vi "Read.vi"(8 "error in (no error)":errorcluster, 11 "Bronkhorst Settings in":T1) -> (0 "error out":errorcluster, 1 "Connection Error":bool, 2 "flow":dbl, 3 "Bronkhorst Settings out":T1)   [LabVIEW 2018, in "Bronkhorst M13 Flow Meter.lvlib"]
uses:
  Bronkhorst M13 Flow Meter.lvlib
  Settings Cluster.ctl
  <vilib>/regexp/Match Regular Expression.xnode
  <vilib>/ptbypt/NI_PtbyPt.lvlib
panel:
  out "x/y":dbl
  out "whole match":string
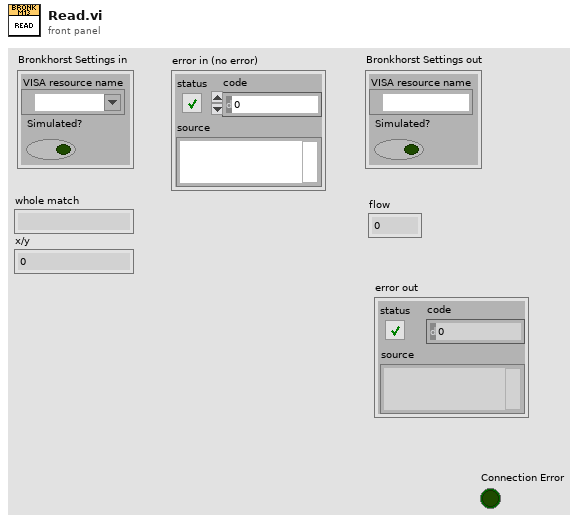
[diagram p1: front panel]
types:
  T1 = typedef "Bronkhorst M13 Flow Meter.lvlib/Settings Cluster.ctl" = cluster{"VISA resource name":refnum<visa-resource-name>, "Simulated?":bool}
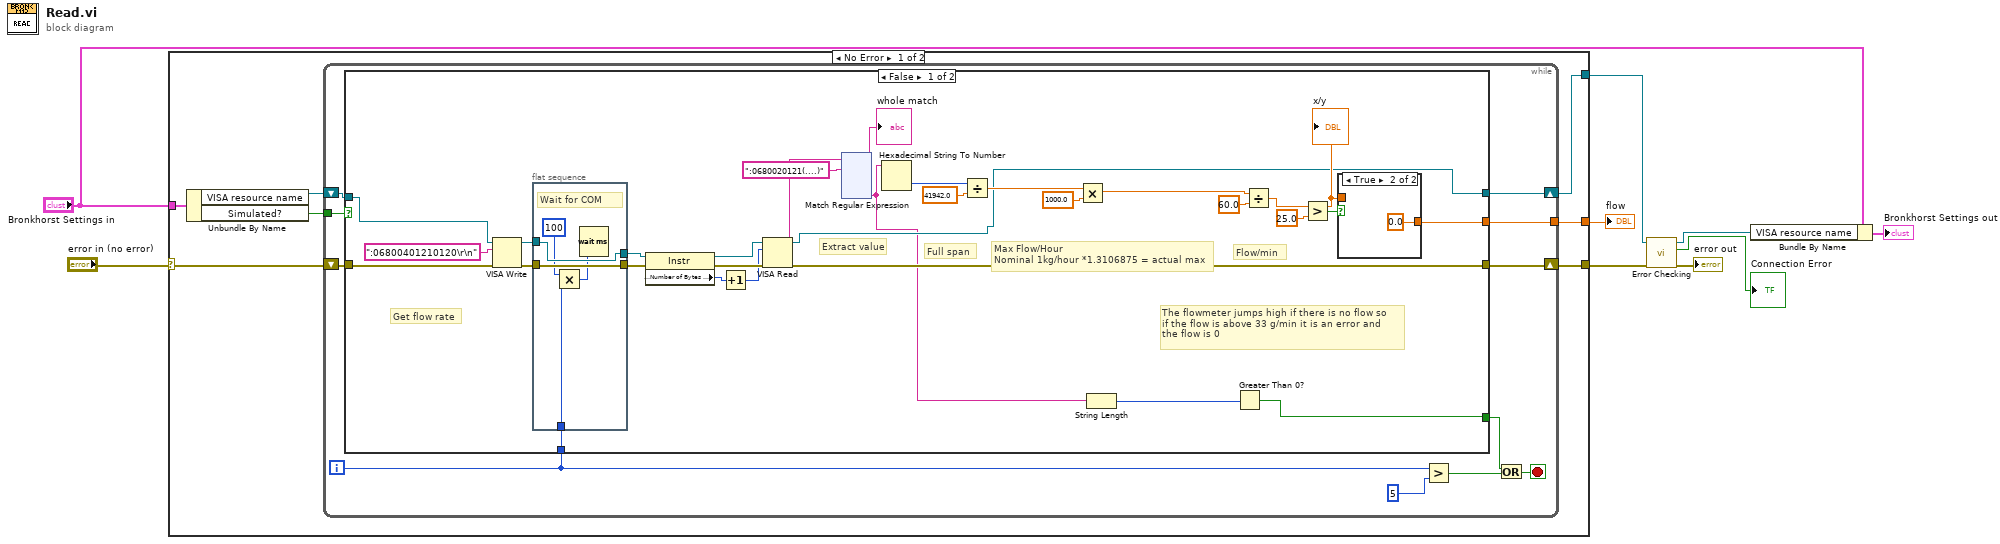
[diagram p0: block diagram]
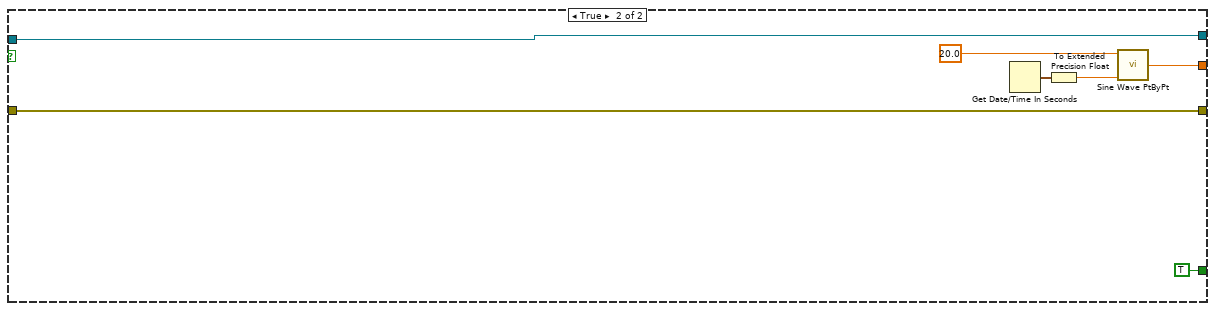
[diagram p3: hidden frame]
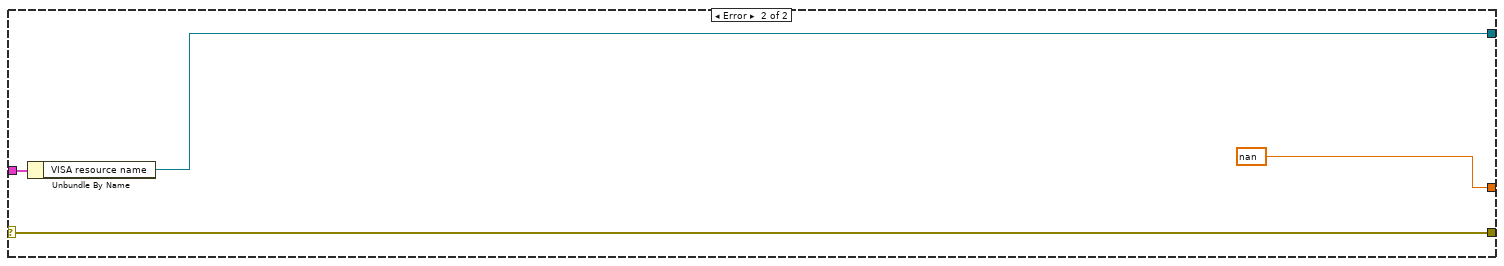
[diagram p4: hidden frame]
diagram:
  n1 = case shown="No Error" "error in (no error)" {
    selector: "error in (no error)" -> [w15 w191]
    tunnel: [w14 w191] -> w3
    tunnel: "Bronkhorst Settings in" -> [w12 w189]
    tunnel: [w13 nan ("sine wave")] -> w9
    tunnel: [w10 w188] -> w5
    frame No Error {
      n2 = Unbundle By Name(w12) -> ("VISA resource name"=w11:refnum<visa-resource-name>, "Simulated?"=w16:bool)
      n3 = while {
        tunnel: w16 -> [w27]
        tunnel: [w24] -> w13
        shift-right: [w25] -> w14
        shift-left: w15 -> [w26]
        shift-right: [w22] -> w10
        shift-left: w11 -> [w23]
        i -> [w18]
        stop <- w17 stop-if-true
        n4 = case shown="False" w27 {
          tunnel: [w33 w187] -> w25
          tunnel: w26 -> [w38 w187]
          tunnel: [w42 w183] -> w24
          tunnel: [w34 w182] -> w22
          tunnel: w23 -> [w39 w182]
          tunnel: [w28 TRUE] -> w19
          tunnel: w18 -> [w30 _]
          frame False {
            # "Flow/min"
            # "Max Flow/Hour\nNominal 1kg/hour *1.3106875 = actual max"
            # "Full span"
            # "Extract value"
            # "Get flow rate"
            # "The flowmeter jumps high if there is no flow so \nif the flow is above 33 g/min it is an error and \nthe flow is 0"
            n5 = VISA Write(VISA resource name=w39, write buffer=":06800401210120\r\n" ("Command"), error in (no error)=w38) -> (VISA resource name out=w54:refnum<visa-resource-name>, error out=w52:errorcluster)  [unwired: 1 out]
            n6 = flat-sequence {
              tunnel: [w180] -> w53
              tunnel: w54 -> [w180]
              tunnel: [w179] -> w51
              tunnel: w52 -> [w179]
              tunnel: w30 -> [w177]
              frame #0 {
                # "Wait for COM"
                n7 = Multiply(x=u32 100 ("milliseconds to wait"), y=w177) -> (x*y=w176:u32)
                n8 = Wait (ms)(milliseconds to wait=w176) -> ()  [unwired: 1 out]
              }
            }
            n9 = property class="Instr"(reference=w53, error in=w51) -> (reference out=w56:refnum<visa-resource-name>, error out=w55:errorcluster, "Serial Settings:Number of Bytes at Serial Port"=w36:u32)
            n10 = Increment(x=w36) -> (x+1=w35:u32)
            n11 = VISA Read(VISA resource name=w56, byte count=w35, error in (no error)=w55) -> (VISA resource name out=w34:refnum<visa-resource-name>, read buffer=w37:string, error out=w33:errorcluster)  [unwired: 1 out]
            n12 = xnode "Match Regular Expression"("input string"=w37, "regular expression"=":0680020121(....)" ("Regular Expression for Extracting Weight")) -> ("whole match"=→"whole match":string, "submatch 1"=w31:string)  [unwired: 4 in, 4 out]
            n13 = Hexadecimal String To Number(string=w31) -> (number=w40:u32)  [unwired: 2 in, 1 out]
            n14 = Divide(x=w40, y=41942.0) -> (x/y=w45:dbl)
            n15 = Multiply(x=w45, y=1000.0) -> (x*y=w32:dbl)
            n16 = String Length(string=w31) -> (length=w29:i32)
            n17 = Greater Than 0?(x=w29) -> (x > 0?=w28:bool)
            n18 = Divide(x=w32, y=60.0) -> (x/y=w43:dbl)
            "x/y" <- w43
            n19 = Greater?(x=w43, y=25.0) -> (0:w44:bool)
            n20 = case shown="True" w44 {
              tunnel: [w58 0.0] -> w42
              tunnel: w43 -> [w58 _]
              frame False {
              }
              frame True {
              }
            }
          }
          frame True {
            n21 = Get Date/Time In Seconds() -> (seconds since 1Jan1904=w186:timestamp)
            n22 = To Extended Precision Float(1:w186) -> (0:w185:ext)
            n23 = call <vilib>:"Sine Wave PtByPt.vi"("time"=w185, "amplitude"=20.0) -> ("sine wave"=w183:dbl)  [unwired: 2 in]
          }
        }
        n24 = Greater?(x=w18, y=5) -> (0:w20:bool)
        n25 = Or(x=w19, y=w20) -> (x .or. y?=w17:bool)
      }
    }
    frame Error {
      n26 = Unbundle By Name(w189) -> ("VISA resource name"=w188:refnum<visa-resource-name>)
    }
  }
  "flow" <- w9
  n27 = call "Error Checking.vi"("error in (no error)"=w3, "VISA resource name"=w5) -> ("error out"=→"error out":errorcluster, "Connection Error"=→"Connection Error":bool, "VISA resource name"=w4:refnum<visa-resource-name>)  [unwired: 7 in]
  n28 = Bundle By Name(cluster="Bronkhorst Settings in", "VISA resource name"=w4) -> (→"Bronkhorst Settings out":T1)
